vi "Open Child.vi"(8 "error in (no error)":errorcluster, 11 "TCP Client in":refnum<class "TCP Client.lvclass">) -> (0 "error out":errorcluster, 3 "TCP Client out":refnum<class "TCP Client.lvclass">)   [LabVIEW 2020, in "Stream-TCP.lvlib" / "TCP Client.lvclass"]
uses:
  TCP Client.lvclass
  Client Command.ctl
  Stream-TCP.lvlib
  lv-stream/stream/Connection/Connection.lvclass
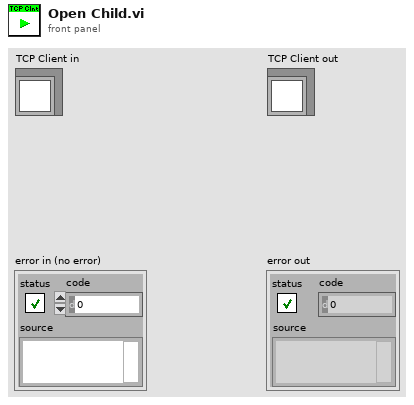
[diagram p1: front panel]
types:
  T1 = typedef "Stream-TCP.lvlib/Client Command.ctl" = enum16{"Connect", "Close", "Shutdown", "Reconnect"}
  T2 = typedef "Stream.lvlib/Connection.lvclass/State.ctl" = enum16{"Closed", "Idle", "Connecting", "Connected", "Shutdown"}
  T3 = typedef "Stream-TCP.lvlib/Client Command Queue.ctl" = refnum<queue>
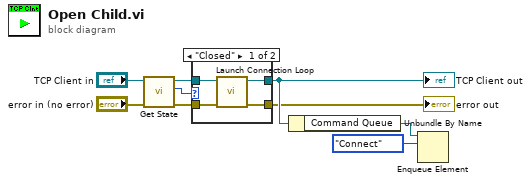
[diagram p0: block diagram]
diagram:
  n1 = call "Get State.vi"("error in (no error)"="error in (no error)", "Connection in"="TCP Client in") -> ("error out"=w1:errorcluster, "State"=w2:T2, "Connection out"=w3:refnum<class "TCP Client.lvclass">)  [unwired: 7 in]
  n2 = case shown="\"Closed\"" w2 {
    tunnel: w3 -> [w13 w15]
    tunnel: w1 -> [w12 w14]
    tunnel: [w11 w15] -> w7
    tunnel: [w10 w14] -> w6
    frame "Closed" {
      n3 = call "Launch Connection Loop.vi"("error in (no error)"=w12, "TCP Client in"=w13) -> ("error out"=w10:errorcluster, "TCP Client out"=w11:refnum<class "TCP Client.lvclass">)  [unwired: 8 in]
    }
    frame Default {
    }
  }
  "error out" <- w6
  "TCP Client out" <- w7
  n4 = Unbundle By Name(w7) -> ("Command Queue"=w9:T3)
  n5 = Enqueue Element(queue=w9, element=Client_Command."Connect") -> ()  [unwired: 2 in, 3 out]
